vi "num to 2 pos.vi"(11 "Motorspeed":dbl) -> (2 "Duty Cycle 2":dbl, 3 "Duty Cycle 1":dbl)   [LabVIEW 2019]
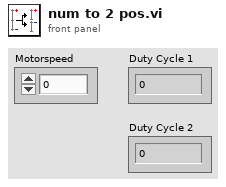
[diagram p1: front panel]
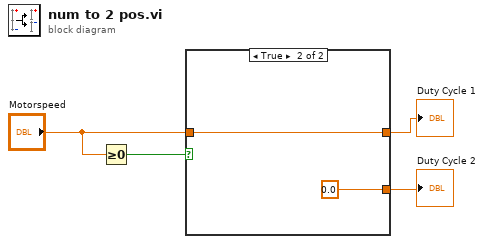
[diagram p0: block diagram]
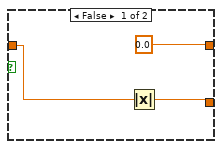
[diagram p2: hidden frame]
diagram:
  n1 = Greater Or Equal To 0?(x="Motorspeed") -> (x >= 0?=w1:bool)
  n2 = case shown="True" w1 {
    tunnel: [w5 0.0] -> w2
    tunnel: [0.0 w8] -> w3
    tunnel: "Motorspeed" -> [w6 w8]
    frame False {
      n3 = Absolute Value(x=w6) -> (abs(x)=w5:dbl)
    }
    frame True {
    }
  }
  "Duty Cycle 2" <- w2
  "Duty Cycle 1" <- w3
